vi "TSM SSC DCPower Filter Sites.vi"(0 "DCPower TSM in":T1, 5 "Requested Sites":i32[](array[numeric]), 11 "error in":errorcluster) -> (4 "Filtered DCPower TSM out":T1, 15 "error out":errorcluster)   [LabVIEW 2019]
doc: "This VI filters the TSM SSC cluster to requested sites."
uses:
  TSM SSC DCPower.ctl
  <vilib>/NI_TestStand_SemiconductorModule/NI_TestStand_Semiconductor_Module.lvlibp/PinMap/PinQueryContext/MultiplePinMultipleSessionQueryContext/MultiplePinMultipleSessionQueryContext.lvclass
  SSC DCPower/SSC DCPower.ctl
  Shared SubVIs/TSM Pin Abstraction/TSM Pin Information.ctl
  Shared SubVIs/TSM Pin Abstraction/TSM Pin Type Identifier.ctl
  Shared SubVIs/TSM Pin Abstraction/TSM Expanded Pin Information.ctl
  Shared SubVIs/Channel List to Pins.vi
  Shared SubVIs/Trim Whitespace [Inlined].vi
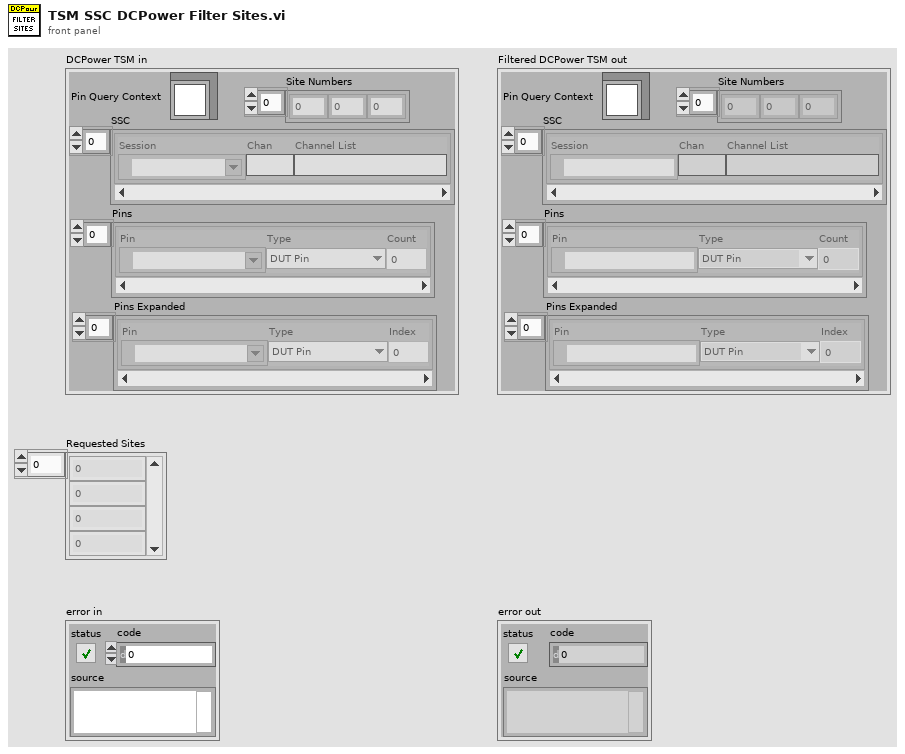
[diagram p1: front panel]
types:
  T1 = typedef "TSM SSC DCPower.ctl" = cluster{"Pin Query Context":refnum<class "MultiplePinMultipleSessionQueryContext.lvclass">, "SSC":T2[], "Site Numbers":i32[], "Pins":T3[], "Pins Expanded":T5[]}
  T2 = typedef "SSC DCPower.ctl" = cluster{"Session":refnum<k15>, "Chan":string, "Channel List":string}
  T3 = typedef "TSM Pin Information.ctl" = cluster{"Pin":tag, "Type":T4, "Count":i32}
  T4 = typedef "TSM Pin Type Identifier.ctl" = enum8{"DUT Pin", "System Pin", "Pin Group", "Not Determined"}
  T5 = typedef "TSM Expanded Pin Information.ctl" = cluster{"Pin":tag, "Type":T4, "Index":i32}
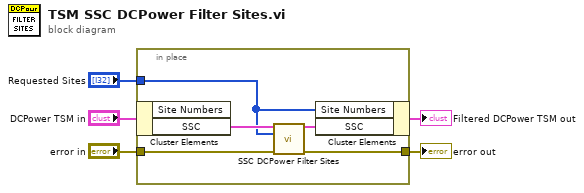
[diagram p0: block diagram]
diagram:
  n1 = in-place {
    in-place-border: "Requested Sites" -> [w8]
    in-place-border: "error in" -> [w7]
    in-place-border: [w6] -> w1
    n2 = in-place-cluster #1("DCPower TSM in") -> ("SSC"=w10:T2[])  [unwired: 1 out]
    n3 = call "SSC DCPower Filter Sites.vi"("DCPower SSC in"=w10, "Requested Sites"=w8, "error in"=w7) -> ("Filtered DCPower SSC out"=w9:T2[], "error out"=w6:errorcluster)  [unwired: 11 in]
    n4 = in-place-cluster #1("Site Numbers"=w8, "SSC"=w9) -> (→"Filtered DCPower TSM out":T1)
  }
  "error out" <- w1
